vi "Set Delay Method (Periodic).vi"(8 "error in (no error)":errorcluster, 9 "Offset":i32, 10 "Range":i32=10 min=10 max=150 step=1, 11 "Abstract Delay Line in":refnum<class "Abstract Delay Line.lvclass">) -> (0 "error out":errorcluster, 3 "Abstract Delay Line out":refnum<class "Abstract Delay Line.lvclass">)   [LabVIEW 2016, in "_Delay Line.lvlib" / "Abstract Delay Line.lvclass"]
uses:
  Abstract Delay Line.lvclass
  Typedef/Delay Method.ctl
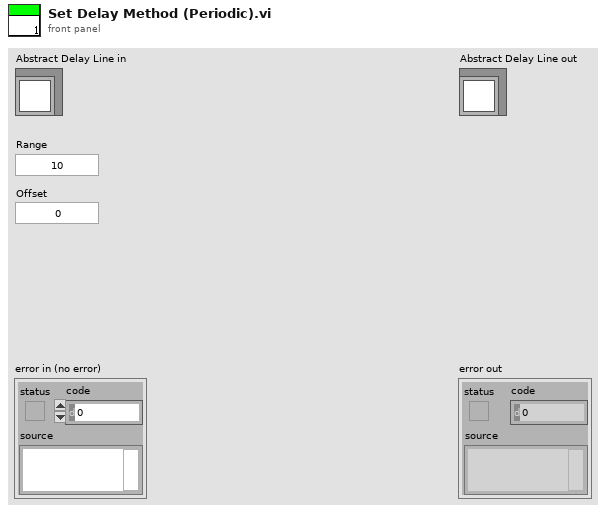
[diagram p1: front panel]
types:
  T1 = typedef "_Delay Line.lvlib/Abstract Delay Line.lvclass/Delay Method.ctl" = enum8{"Periodic", "Fixed"}
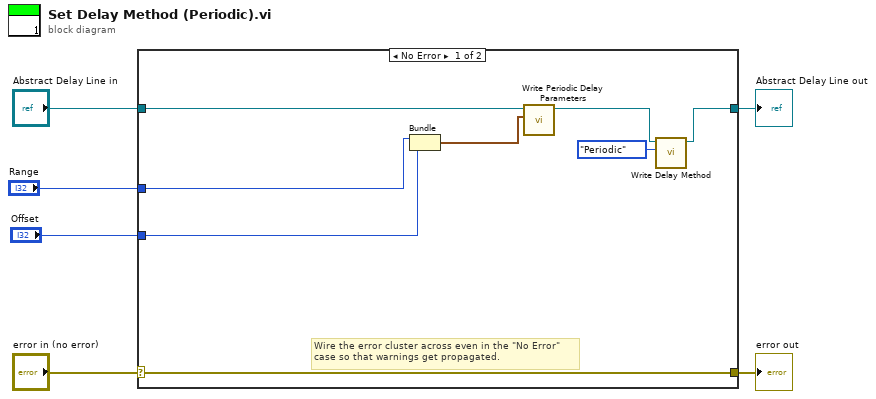
[diagram p0: block diagram]
diagram:
  n1 = case shown="No Error" "error in (no error)" {
    selector: "error in (no error)" -> [w14 w16]
    tunnel: [w14 w16] -> w5
    tunnel: [w8 w15] -> w3
    tunnel: "Abstract Delay Line in" -> [w13 w15]
    tunnel: "Range" -> [w11 _]
    tunnel: "Offset" -> [w10 _]
    frame No Error {
      # "Wire the error cluster across even in the \"No Error\"\ncase so that warnings get propagated."
      n2 = Bundle("Range"=w11, "Offset"=w10) -> (w12:cluster{"Range":i32, "Offset":i32})  [unwired: 1 in]
      n3 = call-dynamic "Write Periodic Delay Parameters.vi"("Periodic Delay Parameters"=w12, "Abstract Delay Line in"=w13) -> ("Abstract Delay Line out"=w9:refnum<class "Abstract Delay Line.lvclass">)  [unwired: 9 in]
      n4 = call-dynamic "Write Delay Method.vi"("Delay Method"=Delay_Method."Periodic", "Abstract Delay Line in"=w9) -> ("Abstract Delay Line out"=w8:refnum<class "Abstract Delay Line.lvclass">)  [unwired: 9 in]
    }
    frame Error {
    }
  }
  "error out" <- w5
  "Abstract Delay Line out" <- w3
